vi "AdjustSamplingTime.vi"(11 "Test Params Cluster":T1={"Test Freq. (Hz)"=1702.3933752476319, "Output Signal Amplitude\nVolts Pk"=0.1, "Sampling Time (s)"=0.01, "Sampling Rate (Hz)"=250000.0, "Output Channel"="Dev3/ao0", "Current Channel"="Dev3/ai1", "Voltage Channel"="Dev3/ai0", "Trigger Channel"="/Dev3/ao/StartTrigger", "Number of runs"=5}) -> (3 "output cluster":T1)   [LabVIEW 2020]
panel:
  out "New sampling time":dbl
  out "Number of samples int periods":dbl
  out "Number of periods":dbl
  out "Num Samples":dbl
  out "Samples Per period":dbl
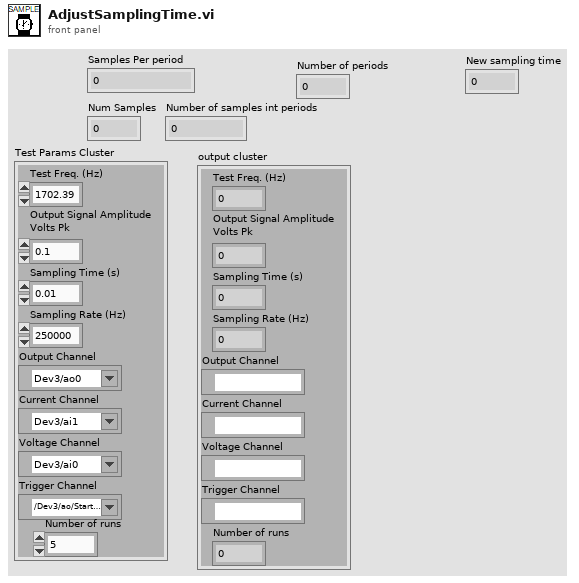
[diagram p1: front panel]
types:
  T1 = cluster{"Test Freq. (Hz)":dbl, "Output Signal Amplitude\nVolts Pk":dbl, "Sampling Time (s)":dbl, "Sampling Rate (Hz)":dbl, "Output Channel":tag, "Current Channel":tag, "Voltage Channel":tag, "Trigger Channel":tag, "Number of runs":i32}
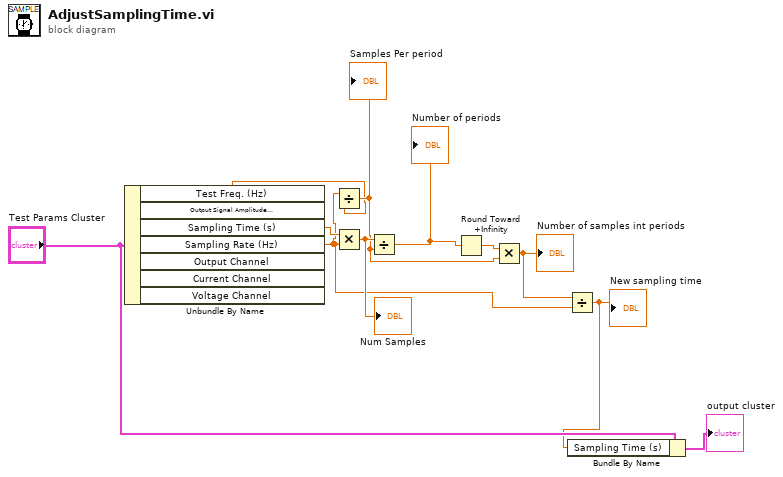
[diagram p0: block diagram]
diagram:
  n1 = Unbundle By Name("Test Params Cluster") -> ("Test Freq. (Hz)"=w4:dbl, "Sampling Time (s)"=w11:dbl, "Sampling Rate (Hz)"=w5:dbl)  [unwired: 4 out]
  n2 = Divide(x=w5, y=w4) -> (x/y=w7:dbl)
  "Samples Per period" <- w7
  n3 = Multiply(x=w11, y=w5) -> (x*y=w10:dbl)
  "Num Samples" <- w10
  n4 = Divide(x=w10, y=w7) -> (x/y=w9:dbl)
  "Number of periods" <- w9
  n5 = Round Toward +Infinity(x=w9) -> (ceil(x): smallest int >= x=w8:dbl)
  n6 = Multiply(x=w8, y=w7) -> (x*y=w6:dbl)
  "Number of samples int periods" <- w6
  n7 = Divide(x=w6, y=w5) -> (x/y=w2:dbl)
  "New sampling time" <- w2
  n8 = Bundle By Name(cluster="Test Params Cluster", "Sampling Time (s)"=w2) -> (→"output cluster":T1)
